vi "Write SubVIs.vi"(5 "SubVIs":refnum<class "SubVI.lvclass">[](array[class]), 9 "Diagram in":refnum<class "Diagram.lvclass">) -> (3 "Diagram out":refnum<class "Diagram.lvclass">)   [LabVIEW 2014, in "Diagram.lvclass"]
uses:
  Diagram.lvclass
  SubVI/SubVI.lvclass
  Diagram.lvclass/Diagram.ctl
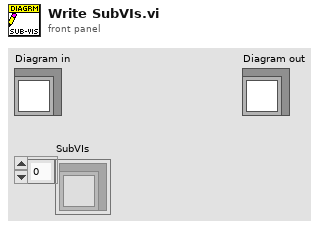
[diagram p1: front panel]
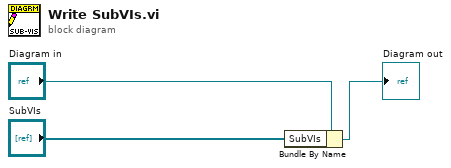
[diagram p0: block diagram]
diagram:
  n1 = Bundle By Name(cluster="Diagram in", "SubVIs"="SubVIs") -> (→"Diagram out":refnum<class "Diagram.lvclass">)
